vi "WaitStop.vi"(8 "error in (no error)":errorcluster, 11 "VISA resource name":refnum<visa-resource-name>) -> (0 "error out":errorcluster, 1 "Com failure Counts":i32, 2 "Moving":bool)   [LabVIEW 2014, in "GRBLMotionCore.lvlib"]
doc: "Performs an instrument error query before terminating the software connection to the instrument."
uses:
  <instrlib>/GRBL/GRBLMotionCore.lvlib
  <instrlib>/GRBL/Public/Position_GRBL.vi
  <vilib>/regexp/Match Regular Expression.xnode
panel:
  out "still?":bool
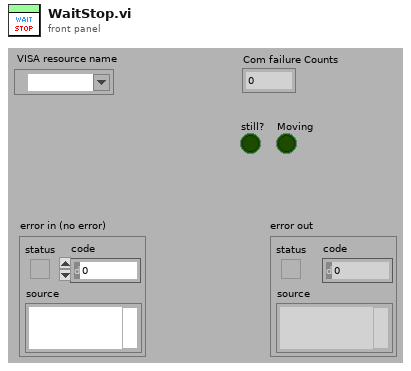
[diagram p1: front panel]
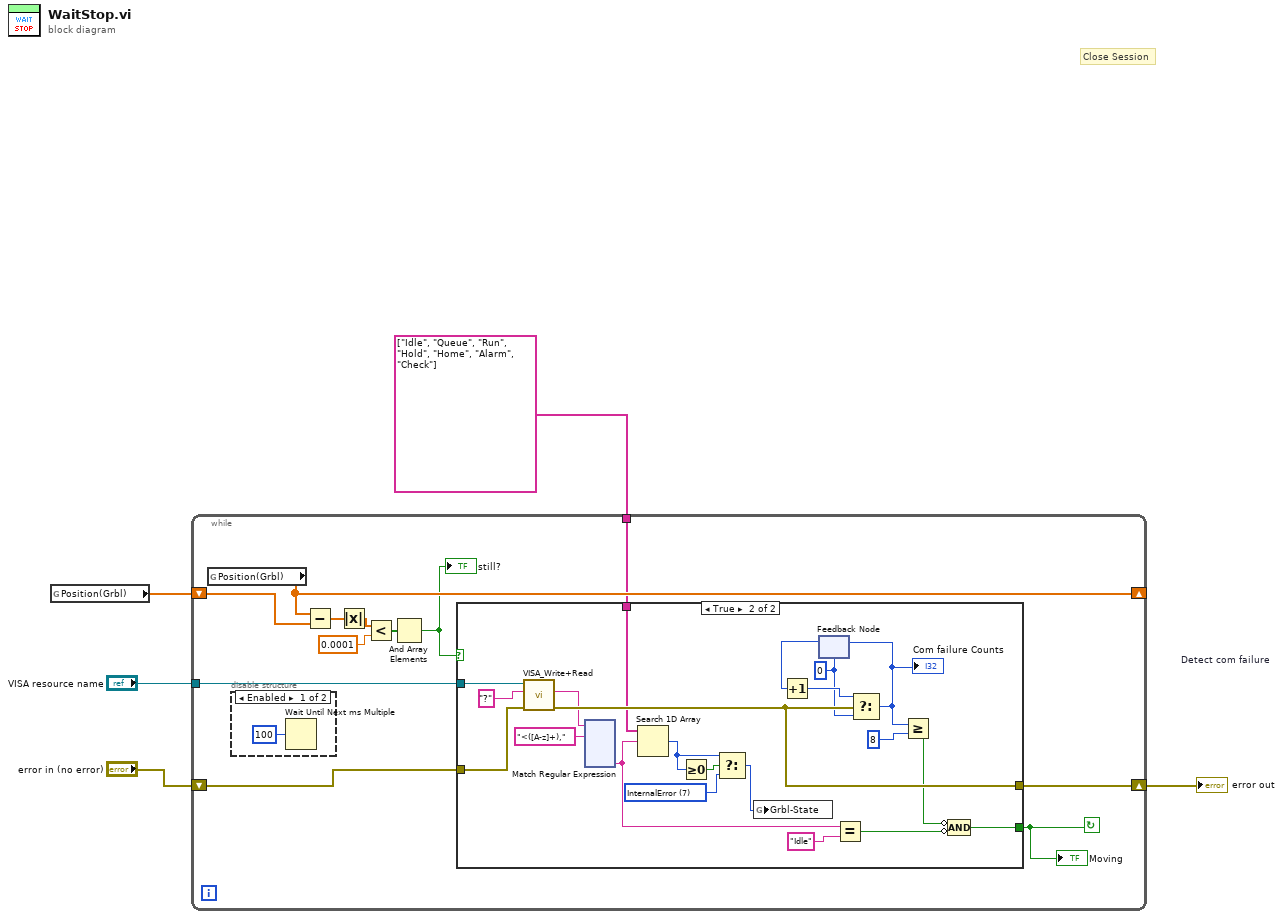
[diagram p0: block diagram]
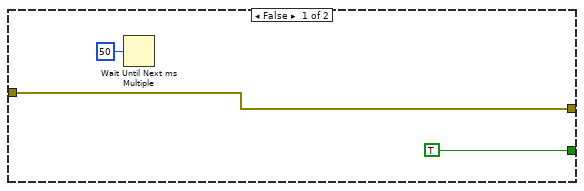
[diagram p3: hidden frame]
diagram:
  # "Close Session"
  n1 = global read "Position_GRBL.vi" "Position(Grbl)"() -> (w2:dbl[])
  n2 = while {
    tunnel: "VISA resource name" -> [w17]
    shift-right: [w16] -> w4
    shift-left: "error in (no error)" -> [w15]
    shift-right: [w14] -> _
    shift-left: w2 -> [w13]
    tunnel: string[] ["Idle", "Queue", "Run", "Hold", "Home", "Alarm", "Check"] ("1D array") -> [w6]
    stop <- w7 continue-if-true
    n3 = global read "Position_GRBL.vi" "Position(Grbl)"() -> (w14:dbl[])
    n4 = disable-structure shown="Enabled" {
      frame Enabled {
        n5 = Wait Until Next ms Multiple(millisecond multiple=u32 100) -> ()  [unwired: 1 out]
      }
      frame Disabled {
      }
    }
    n6 = Subtract(x=w14, y=w13) -> (x-y=w11:dbl[])
    n7 = Absolute Value(x=w11) -> (abs(x)=w8:dbl[])
    n8 = Less?(x=w8, y=0.0001) -> (x < y?=w9:bool[])
    n9 = And Array Elements(Boolean array=w9) -> (logical AND=w12:bool)
    "still?" <- w12
    n10 = case shown="True" w12 {
      tunnel: w17 -> [_ w42]
      tunnel: [w21 w37] -> w16
      tunnel: w15 -> [w21 w41]
      tunnel: [TRUE w40] -> w7
      tunnel: w6 -> [_ w28]
      frame False {
        n11 = Wait Until Next ms Multiple(millisecond multiple=u32 50) -> ()  [unwired: 1 out]
      }
      frame True {
        w25 = 7 items=["Idle", "Queue", "Run", "Hold", "Home", "Alarm", "Check", "InternalError"] ("Grbl-State")
        w34 = 0
        n12 = call <instrlib>:"VISA_Write+Read.vi"("error in (no error)"=w41, "Write Buffer"="?" ("string"), "VISA resource name"=w42) -> ("error out"=w37:errorcluster, "readout"=w29:string)  [unwired: 6 in, 1 out]
        n13 = xnode "Match Regular Expression"("input string"=w29, "regular expression"="<([A-z]+),") -> ("submatch 1"=w27:string)  [unwired: 4 in, 5 out]
        n14 = Search 1D Array(1D array=w28, element=w27) -> (index of element=w22:i32)  [unwired: 1 in]
        n15 = Greater Or Equal To 0?(x=w22) -> (x >= 0?=w24:bool)
        n16 = Select(t=w22, s=w24, f=w25) -> (s? t:f=w23:i32)
        n17 = global write "Position_GRBL.vi" "Grbl-State"(w23) -> ()
        n18 = feedback #1 "Detect com failure"(w34) -> (w35:i32)
        n19 = Increment(x=w35) -> (x+1=w36:i32)
        n20 = Equal?(x=w27, y="Idle") -> (x = y?=w38:bool)
        n21 = Select(t=w36, s=w37, f=w34) -> (s? t:f=w33:i32)
        "Com failure Counts" <- w33
        n22 = feedback-in #1(w33) -> ()
        n23 = Greater Or Equal?(x=w33, y=8) -> (x >= y?=w31:bool)
        n24 = Compound Arithmetic op=AND(invert w31, invert w38) -> (w40:bool)
      }
    }
    "Moving" <- w7
  }
  "error out" <- w4
